vi "practice2_with_strain.vi"() -> ()   [LabVIEW 2014]
doc: "This VI demonstrates the individual configuration of settings in I/W, W/I, and continuous operation modes.\n\nThis VI is not meant to be used with infusion-only models. \n\nNotes:\n(1) If continuous mode is selected, infuse volumes/rates will be used."
uses:
  <instrlib>/KD Scientific 2XX Series/KD Scientific 2XX Series.lvlib
  <vilib>/Motion/FlexMotion/CustomControls/CustomControls.llb/AxisOrVectorSpace To Configure.flx
  <vilib>/Motion/FlexMotion/FunctionsVIs/Trajectory.llb/Check Move Complete Status (8 axes).flx
  <vilib>/Motion/FlexMotion/FunctionsVIs/StartStopMotion.llb/Start Motion (8 axes).flx
  <vilib>/Motion/FlexMotion/FunctionsVIs/StartStopMotion.llb/Stop Motion (8 axes).flx
  <vilib>/vision/NI_Vision_Development_Module.lvlib
panel:
  out "Strain 2 %":dbl
  out "Strain 1 %":dbl
  in  "Distance 2":dbl
  in  "Distance 1":dbl
  out "d 2":i32
  out "d 1":i32
  out "Circle 3":T1
  out "Circle 2":T1
  out "Circle 1":T1
  out "Circles Data (Circle Detection 1)":T2(array[cluster])
  in  "stop (F)":bool
  out "Data from Transducer":dynamicdata(graph) caption="Voltage from Transducer V"
  out "Voltage from pressure transducer":dbl[](array[numeric])
  out "Pressure mm Hg":dbl[](graph)
  in  "Calibration factor":dbl[](array[numeric])
  in  "Zero Error":dbl[](array[numeric])
  out "pressure mm Hg":dbl[](array[numeric])
  in  "stop 2":bool
  out "Voltage (V)":dbl=0.3869919147841388
  out "Force (grams)":dbl=0.3869919147841388
  out "Force Graph (g)":dynamicdata(graph)
  in  "Zero":dbl=-99.6 format="%#_13g"
  out "Load Cell Output (mV)":dynamicdata(graph)
  in  "Displacement in mm":dbl
  in  "Velocity in mm/s":dbl
  out "Image":T3(plugin-control)
  out "Particle Measurements (Pixels) (Particle Analysis 1)":dbl[][](array[numeric]) format="%.2f"
  out "subarray":dbl[](array[numeric])
  out "The diameter":dbl[](array[numeric])
  out "Image from  Vision Acquisition 1":T3(plugin-control)
  out "Units":string
  out "Delivered Volume":dbl
  in  "stop":bool
  out "Status":T4
  in  "Baud Rate (9600)":u32(ring)=9600 items=["300"=300, "1200"=1200, "2400"=2400, "4800"=4800, "9600"=9600]
  in  "Withdrawal Settings":T5={"Flow Rate (5)"=5.0, "Volume (10)"=10.0, "Volume Units (ml)"=enum."milliliters (ml)", "Rate Units (ml/min.)"=enum."milliliters per minute (ml/min.)"} {"Volume (10)" format="%#.3g"}
  in  "Diameter (8.75 mm)":dbl=8.75
  in  "Infusion Settings":T5={"Flow Rate (5)"=5.0, "Volume (10)"=10.0, "Volume Units (ml)"=enum."milliliters (ml)", "Rate Units (ml/min.)"=enum."milliliters per minute (ml/min.)"}
  in  "Operation Mode (Infuse)":u16(ring) items=["Infuse", "Withdraw", "Infuse-Withdraw", "Withdraw-Infuse", "Continuous"]
  in  "Address (0)":i32 format="%0.0f"
  in  "error in (no error)":errorcluster
  in  "VISA resource name":refnum<visa-resource-name>="COM1"
  # "CCD Camera Input"
  # "Load Cell Input"
  # "Syringe Pump Control"
  # "RS-232 Settings"
  # "General Settings"
  # "Pump Status"
  # "Displacement Motor Control"
  # "Pressure Transducer"
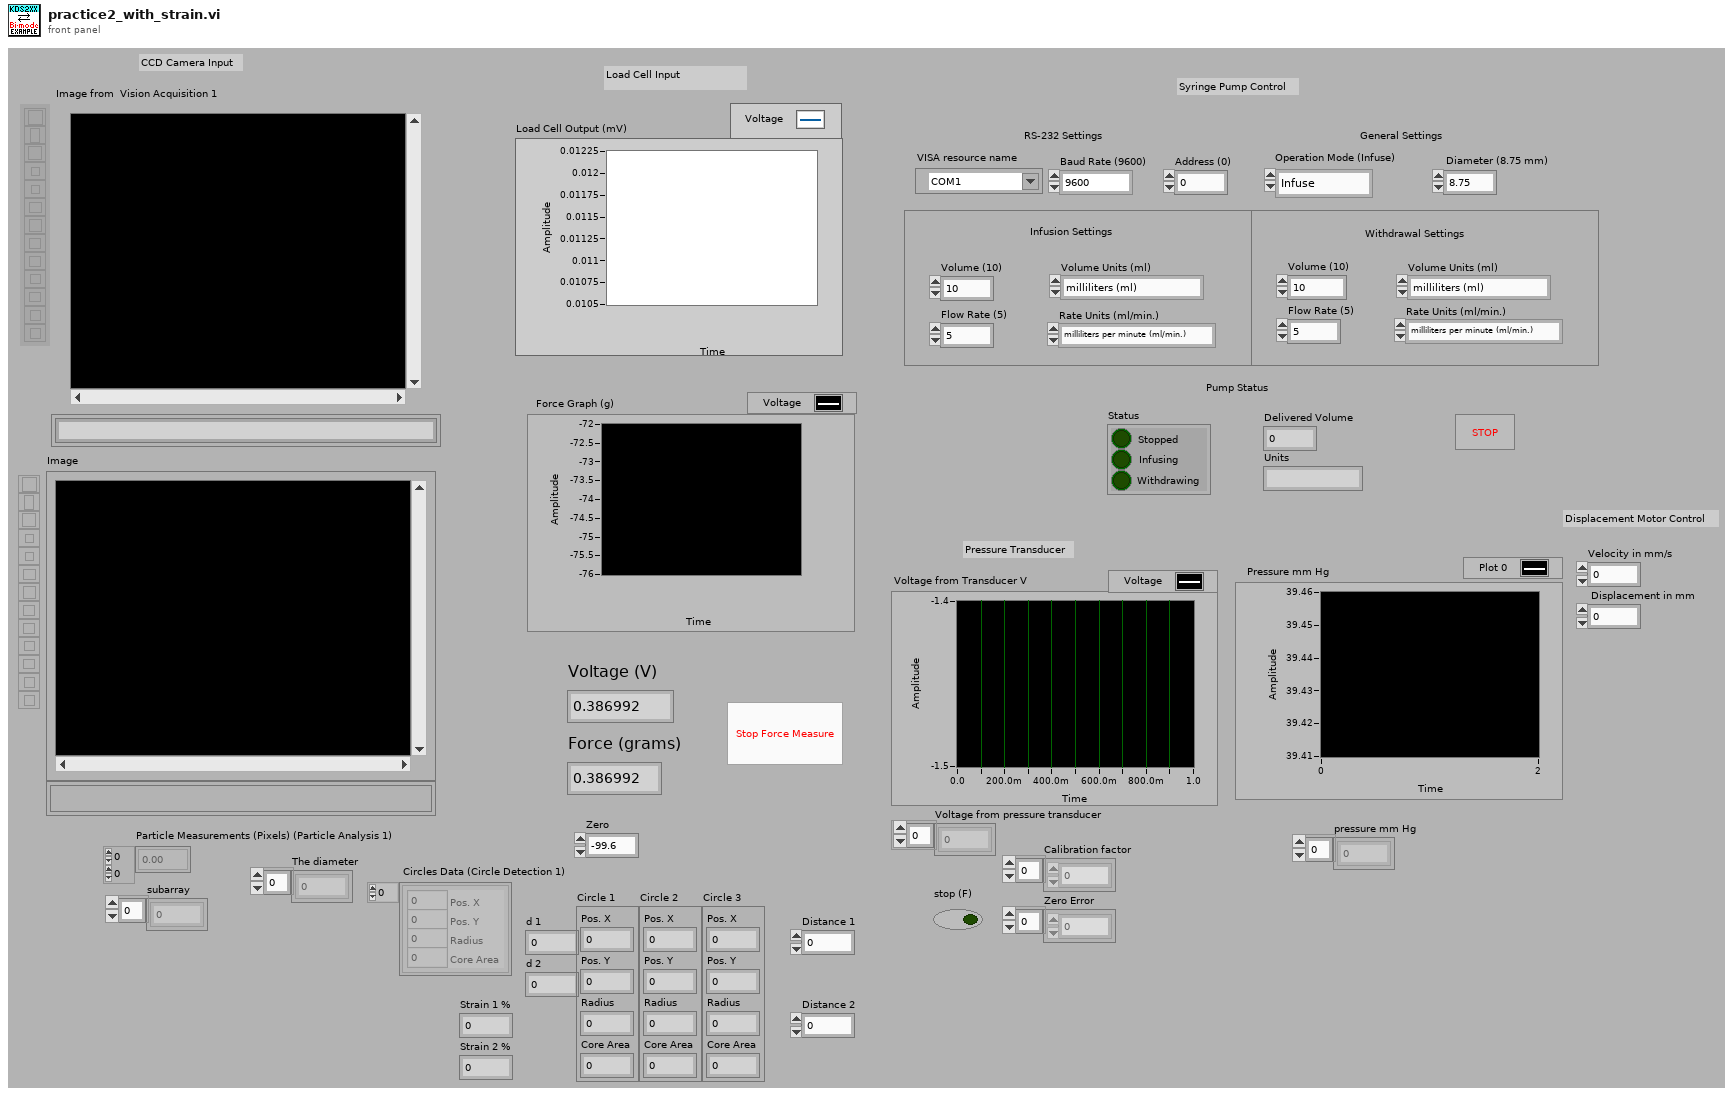
[diagram p1: front panel]
types:
  T1 = cluster{"Pos. X":i32, "Pos. Y":i32, "Radius":i32, "Core Area":i32}
  T2 = cluster{"Pos. X":i32, "Pos. Y":i32, "Radius":i32, "Core Area":i32}[]
  T3 = typedef "IMAQ Image.ctl" = refnum<image>
  T4 = cluster{"Stopped":bool, "Infusing":bool, "Withdrawing":bool}
  T5 = cluster{"Flow Rate (5)":dbl, "Volume (10)":dbl, "Volume Units (ml)":enum16{"milliliters (ml)", "microliters (ul)"}, "Rate Units (ml/min.)":enum16{"milliliters per minute (ml/min.)", "milliliters per hour (ml/hr.)", "microliters per minute (ul/min.)", "microliters per hour (ul/hr.)"}}
  T6 = typedef "Board Id" = u8
  T7 = enum16{"Absolute Position", "Relative Position", "Velocity", "Relative to Cap Pos", "Modulus Position", "Absolute Contouring", "Relative Contouring"}
  T8 = typedef "ROI Descriptor" = cluster{"Global Rectangle":i32[], "Contours":cluster{"ID":enum32{"External", "Internal"}, "Type":u32, "Coordinates":i32[]}[]}
  T9 = typedef "AxisOrVectorSpace To Configure.flx" = u16
  T10 = typedef "Resource Out (Enum).flx" = u16
  T11 = typedef "Bd Id Out" = u8
  T12 = enum16{"milliliters per minute (ml/min.)", "milliliters per hour (ml/hr.)", "microliters per minute (ul/min.)", "microliters per hour (ul/hr.)"}
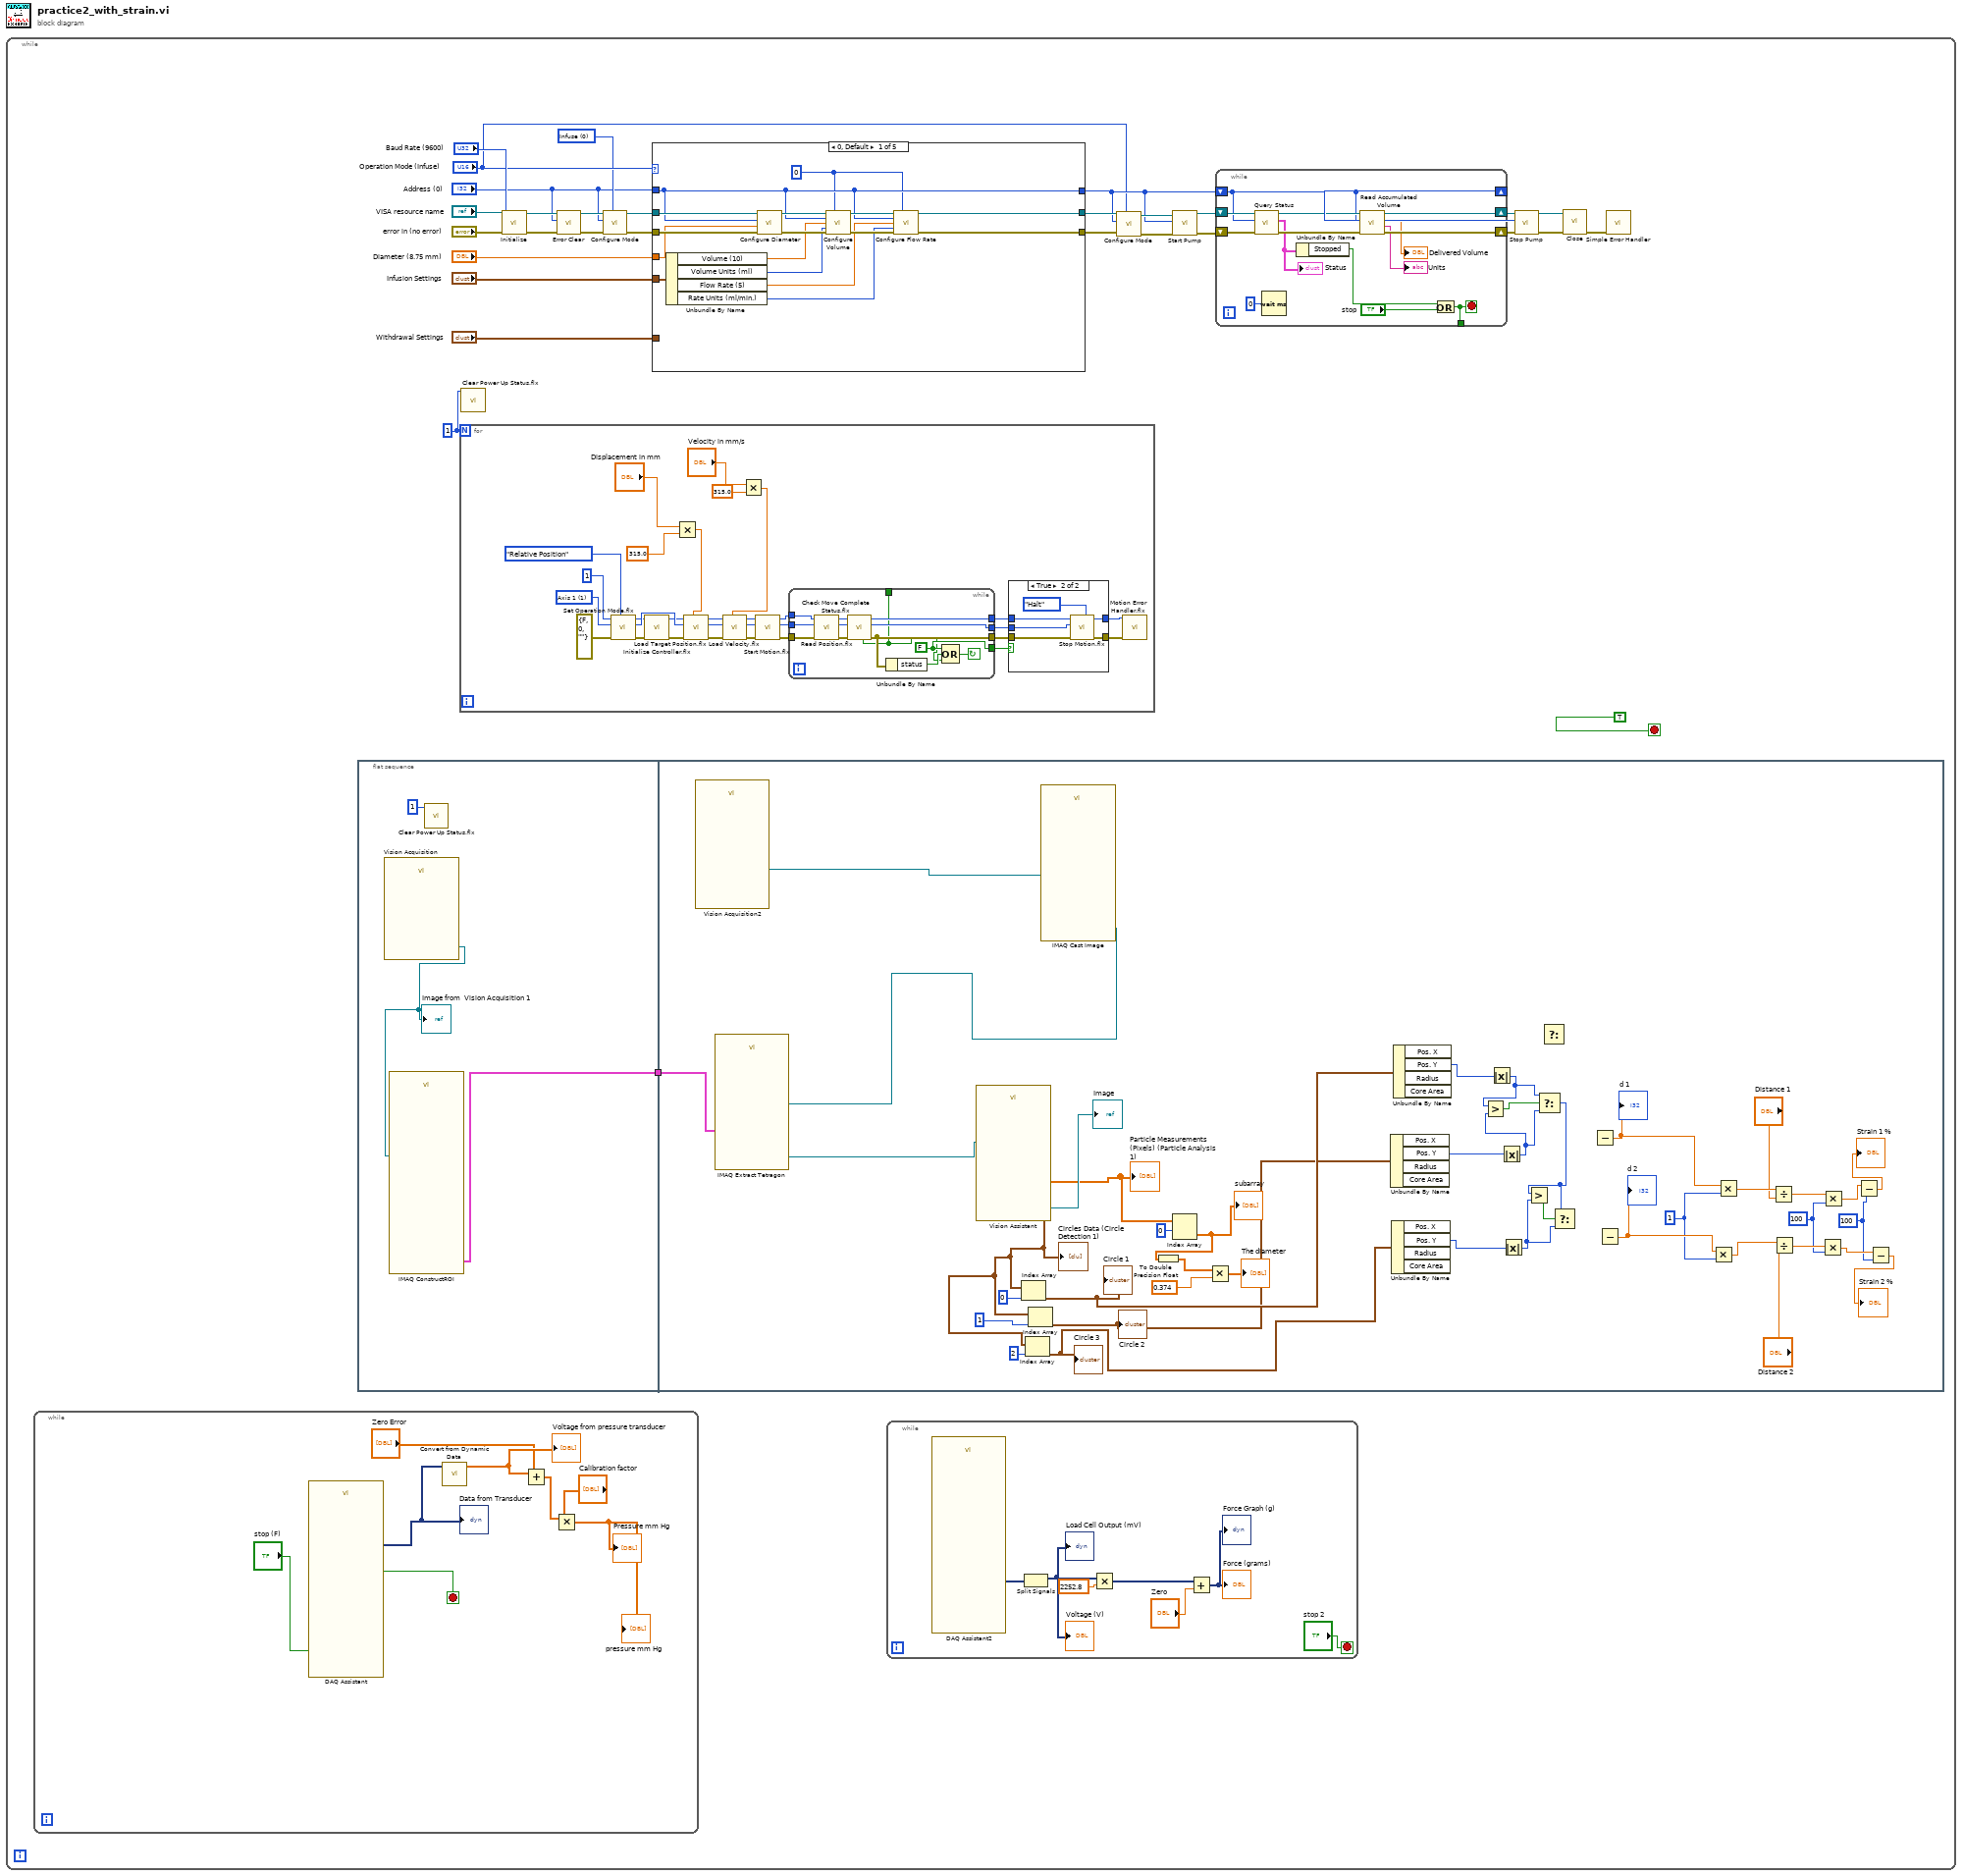
[diagram p0: block diagram]
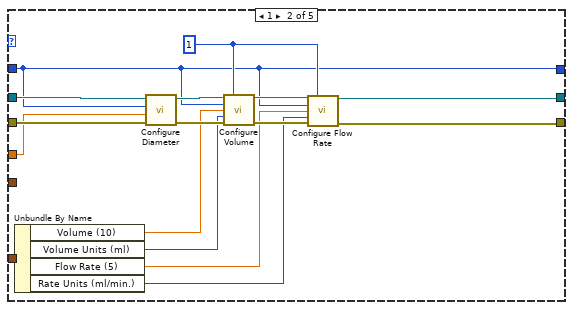
[diagram p3: hidden frame]
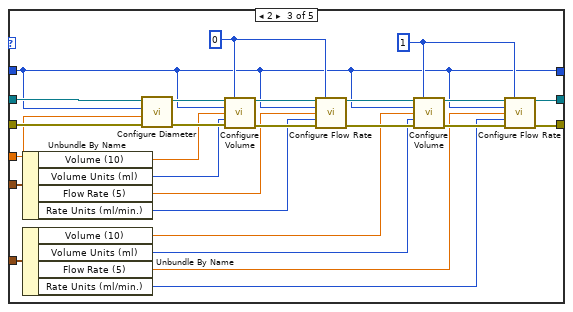
[diagram p4: hidden frame]
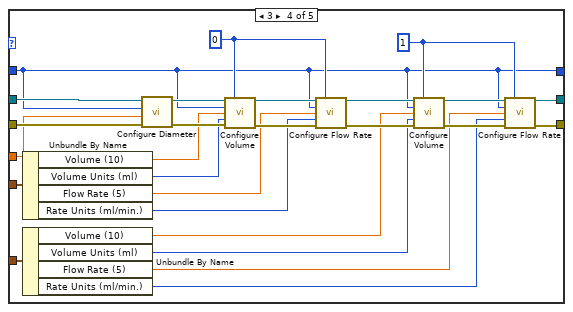
[diagram p5: hidden frame]
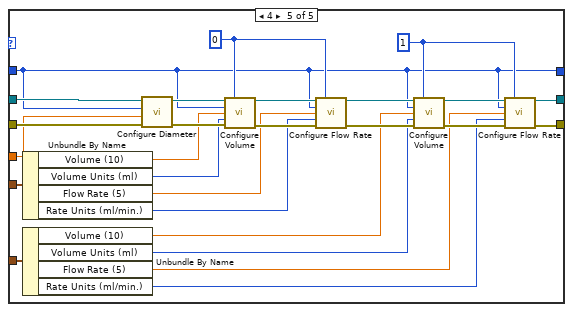
[diagram p6: hidden frame]
diagram:
  n1 = while {
    stop <- TRUE stop-if-true
    w3 = T6 1 ("Board ID")
    w9 = u16 0 items=["Infuse", "Withdraw", "Infuse-Withdraw", "Withdraw-Infuse", "Continuous"] ("Mode (infuse)")
    n2 = flat-sequence {
      tunnel: [w41] -> w1
      tunnel: w1 -> [w83]
      frame #0 {
        n3 = call "Vision Acquisition"() -> ("Image Out"=w39:T3)  [unwired: 26 in, 1 out]
        "Image from  Vision Acquisition 1" <- w39
        n4 = call "IMAQ ConstructROI"("Image"=w39) -> ("ROI Descriptor Out"=w41:T8)  [unwired: 7 in, 3 out]
        n5 = call <vilib>:"Clear Power Up Status.flx"("Board ID"=T6 1) -> ()  [unwired: 6 in, 2 out]
      }
      frame #1 {
        w53 = 100
        w56 = 100
        w63 = 1
        n6 = call "Vision Acquisition2"() -> ("Image Out"=w81:T3)  [unwired: 25 in, 2 out]
        n7 = call "IMAQ Cast Image"("Image Src"=w81) -> ("Image Dst Out"=w80:T3)  [unwired: 9 in, 1 out]
        n8 = call-poly "IMAQ Extract Tetragon"("ROI Descriptor"=w83, "Image Src"=w80) -> ("Image Dst Out"=w73:T3)  [unwired: 8 in, 1 out]
        n9 = call "Vision Assistant"("Image In"=w73) -> ("Image Out"=→"Image":T3, "Particle Measurements (Pixels) (Particle Analysis 1)"=w79:dbl[][], "Circles Data (Circle Detection 1)"=w70:T2)  [unwired: 22 in, 2 out]
        "Particle Measurements (Pixels) (Particle Analysis 1)" <- w79
        "Circles Data (Circle Detection 1)" <- w70
        n10 = Index Array(array=w70, index=0) -> (element=w68:T1)
        "Circle 1" <- w68
        n11 = Index Array(array=w70, index=2) -> (element=w66:T1)
        "Circle 3" <- w66
        n12 = Index Array(array=w70, index=1) -> (element=w67:T1)
        "Circle 2" <- w67
        n13 = Index Array(array=w79, index (row)=0) -> (element=w77:dbl[])  [unwired: 1 in]
        "subarray" <- w77
        n14 = To Double Precision Float(number=w77) -> (double precision float=w76:dbl[])
        n15 = Multiply(x=w76, y=0.374) -> (x*y=→"The diameter":dbl[])
        n16 = Unbundle By Name(w67) -> ("Pos. Y"=w49:i32)  [unwired: 3 out]
        n17 = Unbundle By Name(w66) -> ("Pos. Y"=w48:i32)  [unwired: 3 out]
        n18 = Unbundle By Name(w68) -> ("Pos. Y"=w50:i32)  [unwired: 3 out]
        n19 = Absolute Value(x=w50) -> (abs(x)=w46:i32)
        n20 = Absolute Value(x=w49) -> (abs(x)=w45:i32)
        n21 = Greater?(x=w46, y=w45) -> (0:w47:bool)
        n22 = Absolute Value(x=w48) -> (abs(x)=w42:i32)
        n23 = Select(t=w46, s=w47, f=w45) -> (s? t:f=w43:i32)
        n24 = Greater?(x=w43, y=w42) -> (0:w44:bool)
        n25 = Select() -> ()  [unwired: 3 in, 1 out]
        n26 = Select(t=w43, s=w44, f=w42) -> ()  [unwired: 1 out]
        n27 = Subtract() -> (x-y=w65:dbl)  [unwired: 2 in]
        "d 1" <- w65
        n28 = Subtract() -> (x-y=w64:dbl)  [unwired: 2 in]
        "d 2" <- w64
        n29 = Multiply(x=w64, y=w63) -> (x*y=w61:dbl)
        n30 = Multiply(x=w65, y=w63) -> (x*y=w62:dbl)
        n31 = Divide(x=w62, y="Distance 1") -> (x/y=w58:dbl)
        n32 = Divide(x=w61, y="Distance 2") -> (x/y=w57:dbl)
        n33 = Multiply(x=w57, y=w56) -> (x*y=w54:dbl)
        n34 = Multiply(x=w58, y=w56) -> (x*y=w55:dbl)
        n35 = Subtract(x=w55, y=w53) -> (x-y=→"Strain 1 %":dbl)
        n36 = Subtract(x=w54, y=w53) -> (x-y=→"Strain 2 %":dbl)
      }
    }
    n37 = for {
      N: w3 -> [_]
      w111 = T9 1 items=["Axis 1"=1, "Axis 2"=2, "Axis 3"=3, "Axis 4"=4, "Axis 5"=5, "Axis 6"=6, "Axis 7"=7, "Axis 8"=8, "Vector Space 1"=17, "Vector Space 2"=18, "Vector Space 3"=19, "Vector Space 4"=20] ("Axis or Vector Space")
      n38 = call <vilib>:"Set Operation Mode.flx"("Position Mode (Absolute)"=T7."Relative Position", "error in (no error)"=errorcluster {"status"=FALSE, "code"=0, "source"=""} ("error constant"), "Axis or Vector Space"=w111, "Board ID"=T6 1) -> ("error out"=w109:errorcluster, "Resource Output"=w108:T10, "Bd ID Out"=w107:T11)  [unwired: 2 in]
      n39 = call <vilib>:"Initialize Controller.flx"("error in (no error)"=w109, "Board ID"=w107) -> ("error out"=w102:errorcluster, "Bd ID Out"=w106:T11)  [unwired: 6 in]
      n40 = Multiply(x="Displacement in mm", y=315.0) -> (x*y=w86:dbl)
      n41 = call <vilib>:"Load Target Position.flx"("Target Position (0)"=w86, "error in (no error)"=w102, "Axis"=w108, "Board ID"=w106) -> ("error out"=w103:errorcluster, "Resource Output"=w104:T10, "Bd ID Out"=w105:T11)  [unwired: 3 in]
      n42 = Multiply(x="Velocity in mm/s", y=315.0) -> (x*y=w87:dbl)
      n43 = call <vilib>:"Load Velocity.flx"("Velocity (10000)"=w87, "error in (no error)"=w103, "Axis or Vector Space"=w104, "Board ID"=w105) -> ("error out"=w99:errorcluster, "Resource Output"=w100:T10, "Bd ID Out"=w101:T11)  [unwired: 3 in]
      n44 = call-poly <vilib>:"Start Motion.flx"("error in (no error)"=w99, "Axis or Vector Space"=w100, "Board ID"=w101) -> ("error out"=w96:errorcluster, "Resource Output"=w97:T10, "Bd ID Out"=w98:T11)  [unwired: 3 in]
      n45 = while {
        tunnel: w98 -> [w134]
        tunnel: w97 -> [w133]
        tunnel: w96 -> [w132]
        tunnel: [w127] -> w95
        tunnel: [w126] -> w94
        tunnel: [w124] -> w93
        tunnel: [w123] -> w92
        tunnel: [w122] -> _
        stop <- w128 continue-if-true
        w127 = FALSE
        n46 = call <vilib>:"Read Position.flx"("error in (no error)"=w132, "Axis"=w133, "Board ID"=w134) -> ("error out"=w129:errorcluster, "Resource Output"=w130:T10, "Bd ID Out"=w131:T11)  [unwired: 3 in, 1 out]
        n47 = call-poly <vilib>:"Check Move Complete Status.flx"("error in (no error)"=w129, "Axis or Vector Space"=w130, "Board ID"=w131) -> ("error out"=w126:errorcluster, "Resource Output"=w123:T10, "Bd ID Out"=w124:T11, "Move Complete"=w122:bool)  [unwired: 3 in]
        n48 = Unbundle By Name(w126) -> ("status"=w125:bool)
        n49 = Compound Arithmetic op=OR(w127, w125, w122) -> (w128:bool)
      }
      n50 = case shown="True" w95 {
        tunnel: w94 -> [w114 w120]
        tunnel: w93 -> [w115 w119]
        tunnel: w92 -> [_ w118]
        tunnel: [w114 w117] -> w91
        tunnel: [w115 w116] -> w90
        frame False {
        }
        frame True {
          n51 = call-poly <vilib>:"Stop Motion.flx"("Stop Type (Decel)"=enum16{"Decelerate", "Halt", "Kill"}."Halt", "error in (no error)"=w120, "Axis or Vector Space"=w118, "Board ID"=w119) -> ("error out"=w117:errorcluster, "Bd ID Out"=w116:T11)  [unwired: 3 in, 1 out]
        }
      }
      n52 = call <vilib>:"Motion Error Handler.flx"("Board ID"=w90, "error in (no error)"=w91) -> ()  [unwired: 9 in, 5 out]
    }
    n53 = call <vilib>:"Clear Power Up Status.flx"("Board ID"=w3) -> ()  [unwired: 6 in, 2 out]
    n54 = call <instrlib>:"Initialize.vi"("error in (no error)"="error in (no error)", "Baud Rate (9600)"="Baud Rate (9600)", "VISA resource name"="VISA resource name") -> ("error out"=w6:errorcluster, "VISA resource name out"=w5:refnum<visa-resource-name>)  [unwired: 7 in]
    n55 = call <instrlib>:"Error Clear.vi"("error in (no error)"=w6, "Address (0)"="Address (0)", "VISA resource name"=w5) -> ("error out"=w7:errorcluster, "VISA resource name out"=w8:refnum<visa-resource-name>)  [unwired: 6 in, 1 out]
    n56 = call <instrlib>:"Configure Mode.vi"("Mode (infuse)"=w9, "error in (no error)"=w7, "Address (0)"="Address (0)", "VISA resource name"=w8) -> ("error out"=w11:errorcluster, "VISA resource name out"=w10:refnum<visa-resource-name>)  [unwired: 6 in]
    n57 = case shown="0, Default" "Operation Mode (Infuse)" {
      tunnel: "Infusion Settings" -> [w144 _ w192 w218 w244]
      tunnel: "Withdrawal Settings" -> [_ w166 w191 w217 w243]
      tunnel: w10 -> [w150 w165 w190 w216 w242]
      tunnel: w11 -> [w149 w161 w189 w215 w241]
      tunnel: "Diameter (8.75 mm)" -> [w143 w157 w172 w198 w224]
      tunnel: [w142 w151 w167 w193 w219] -> w13
      tunnel: "Address (0)" -> [w142 w151 w167 w193 w219]
      tunnel: [w137 w162 w169 w195 w221] -> w17
      tunnel: [w136 w158 w168 w194 w220] -> w16
      frame 0, Default {
        w135 = 0
        n58 = Unbundle By Name(w144) -> ("Volume (10)"=w141:dbl, "Volume Units (ml)"=w140:enum16{"milliliters (ml)", "microliters (ul)"}, "Flow Rate (5)"=w139:dbl, "Rate Units (ml/min.)"=w138:T12)
        n59 = call <instrlib>:"Configure Diameter.vi"("error in (no error)"=w149, "Diameter (8.75 mm)"=w143, "Address (0)"=w142, "VISA resource name"=w150) -> ("error out"=w147:errorcluster, "VISA resource name out"=w148:refnum<visa-resource-name>)  [unwired: 6 in]
        n60 = call <instrlib>:"Configure Volume.vi"("VISA resource name"=w148, "Mode (infuse)"=w135, "Address (0)"=w142, "Volume (100)"=w141, "Units (0: milliliters)"=w140, "error in (no error)"=w147) -> ("VISA resource name out"=w146:refnum<visa-resource-name>, "error out"=w145:errorcluster)  [unwired: 8 in]
        n61 = call <instrlib>:"Configure Flow Rate.vi"("VISA resource name"=w146, "Mode (infuse)"=w135, "Address (0)"=w142, "Flow Rate (5)"=w139, "Units (0: milliliters per minute)"=w138, "error in (no error)"=w145) -> ("VISA resource name out"=w137:refnum<visa-resource-name>, "error out"=w136:errorcluster)  [unwired: 8 in]
      }
      frame 1 {
        w152 = 1
        n62 = Unbundle By Name(w166) -> ("Volume (10)"=w156:dbl, "Volume Units (ml)"=w155:enum16{"milliliters (ml)", "microliters (ul)"}, "Flow Rate (5)"=w154:dbl, "Rate Units (ml/min.)"=w153:T12)
        n63 = call <instrlib>:"Configure Diameter.vi"("error in (no error)"=w161, "Diameter (8.75 mm)"=w157, "Address (0)"=w151, "VISA resource name"=w165) -> ("error out"=w160:errorcluster, "VISA resource name out"=w164:refnum<visa-resource-name>)  [unwired: 6 in]
        n64 = call <instrlib>:"Configure Volume.vi"("VISA resource name"=w164, "Mode (infuse)"=w152, "Address (0)"=w151, "Volume (100)"=w156, "Units (0: milliliters)"=w155, "error in (no error)"=w160) -> ("VISA resource name out"=w163:refnum<visa-resource-name>, "error out"=w159:errorcluster)  [unwired: 8 in]
        n65 = call <instrlib>:"Configure Flow Rate.vi"("VISA resource name"=w163, "Mode (infuse)"=w152, "Address (0)"=w151, "Flow Rate (5)"=w154, "Units (0: milliliters per minute)"=w153, "error in (no error)"=w159) -> ("VISA resource name out"=w162:refnum<visa-resource-name>, "error out"=w158:errorcluster)  [unwired: 8 in]
      }
      frame 2 {
        w170 = 1
        w171 = 0
        n66 = Unbundle By Name(w192) -> ("Volume (10)"=w180:dbl, "Volume Units (ml)"=w179:enum16{"milliliters (ml)", "microliters (ul)"}, "Flow Rate (5)"=w178:dbl, "Rate Units (ml/min.)"=w177:T12)
        n67 = Unbundle By Name(w191) -> ("Volume (10)"=w176:dbl, "Volume Units (ml)"=w175:enum16{"milliliters (ml)", "microliters (ul)"}, "Flow Rate (5)"=w174:dbl, "Rate Units (ml/min.)"=w173:T12)
        n68 = call <instrlib>:"Configure Diameter.vi"("error in (no error)"=w189, "Diameter (8.75 mm)"=w172, "Address (0)"=w167, "VISA resource name"=w190) -> ("error out"=w184:errorcluster, "VISA resource name out"=w188:refnum<visa-resource-name>)  [unwired: 6 in]
        n69 = call <instrlib>:"Configure Volume.vi"("VISA resource name"=w188, "Mode (infuse)"=w171, "Address (0)"=w167, "Volume (100)"=w180, "Units (0: milliliters)"=w179, "error in (no error)"=w184) -> ("VISA resource name out"=w187:refnum<visa-resource-name>, "error out"=w183:errorcluster)  [unwired: 8 in]
        n70 = call <instrlib>:"Configure Flow Rate.vi"("VISA resource name"=w187, "Mode (infuse)"=w171, "Address (0)"=w167, "Flow Rate (5)"=w178, "Units (0: milliliters per minute)"=w177, "error in (no error)"=w183) -> ("VISA resource name out"=w186:refnum<visa-resource-name>, "error out"=w182:errorcluster)  [unwired: 8 in]
        n71 = call <instrlib>:"Configure Volume.vi"("VISA resource name"=w186, "Mode (infuse)"=w170, "Address (0)"=w167, "Volume (100)"=w176, "Units (0: milliliters)"=w175, "error in (no error)"=w182) -> ("VISA resource name out"=w185:refnum<visa-resource-name>, "error out"=w181:errorcluster)  [unwired: 8 in]
        n72 = call <instrlib>:"Configure Flow Rate.vi"("VISA resource name"=w185, "Mode (infuse)"=w170, "Address (0)"=w167, "Flow Rate (5)"=w174, "Units (0: milliliters per minute)"=w173, "error in (no error)"=w181) -> ("VISA resource name out"=w169:refnum<visa-resource-name>, "error out"=w168:errorcluster)  [unwired: 8 in]
      }
      frame 3 {
        w196 = 1
        w197 = 0
        n73 = Unbundle By Name(w218) -> ("Volume (10)"=w206:dbl, "Volume Units (ml)"=w205:enum16{"milliliters (ml)", "microliters (ul)"}, "Flow Rate (5)"=w204:dbl, "Rate Units (ml/min.)"=w203:T12)
        n74 = Unbundle By Name(w217) -> ("Volume (10)"=w202:dbl, "Volume Units (ml)"=w201:enum16{"milliliters (ml)", "microliters (ul)"}, "Flow Rate (5)"=w200:dbl, "Rate Units (ml/min.)"=w199:T12)
        n75 = call <instrlib>:"Configure Diameter.vi"("error in (no error)"=w215, "Diameter (8.75 mm)"=w198, "Address (0)"=w193, "VISA resource name"=w216) -> ("error out"=w210:errorcluster, "VISA resource name out"=w214:refnum<visa-resource-name>)  [unwired: 6 in]
        n76 = call <instrlib>:"Configure Volume.vi"("VISA resource name"=w214, "Mode (infuse)"=w197, "Address (0)"=w193, "Volume (100)"=w206, "Units (0: milliliters)"=w205, "error in (no error)"=w210) -> ("VISA resource name out"=w213:refnum<visa-resource-name>, "error out"=w209:errorcluster)  [unwired: 8 in]
        n77 = call <instrlib>:"Configure Flow Rate.vi"("VISA resource name"=w213, "Mode (infuse)"=w197, "Address (0)"=w193, "Flow Rate (5)"=w204, "Units (0: milliliters per minute)"=w203, "error in (no error)"=w209) -> ("VISA resource name out"=w212:refnum<visa-resource-name>, "error out"=w208:errorcluster)  [unwired: 8 in]
        n78 = call <instrlib>:"Configure Volume.vi"("VISA resource name"=w212, "Mode (infuse)"=w196, "Address (0)"=w193, "Volume (100)"=w202, "Units (0: milliliters)"=w201, "error in (no error)"=w208) -> ("VISA resource name out"=w211:refnum<visa-resource-name>, "error out"=w207:errorcluster)  [unwired: 8 in]
        n79 = call <instrlib>:"Configure Flow Rate.vi"("VISA resource name"=w211, "Mode (infuse)"=w196, "Address (0)"=w193, "Flow Rate (5)"=w200, "Units (0: milliliters per minute)"=w199, "error in (no error)"=w207) -> ("VISA resource name out"=w195:refnum<visa-resource-name>, "error out"=w194:errorcluster)  [unwired: 8 in]
      }
      frame 4 {
        w222 = 1
        w223 = 0
        n80 = Unbundle By Name(w244) -> ("Volume (10)"=w232:dbl, "Volume Units (ml)"=w231:enum16{"milliliters (ml)", "microliters (ul)"}, "Flow Rate (5)"=w230:dbl, "Rate Units (ml/min.)"=w229:T12)
        n81 = Unbundle By Name(w243) -> ("Volume (10)"=w228:dbl, "Volume Units (ml)"=w227:enum16{"milliliters (ml)", "microliters (ul)"}, "Flow Rate (5)"=w226:dbl, "Rate Units (ml/min.)"=w225:T12)
        n82 = call <instrlib>:"Configure Diameter.vi"("error in (no error)"=w241, "Diameter (8.75 mm)"=w224, "Address (0)"=w219, "VISA resource name"=w242) -> ("error out"=w236:errorcluster, "VISA resource name out"=w240:refnum<visa-resource-name>)  [unwired: 6 in]
        n83 = call <instrlib>:"Configure Volume.vi"("VISA resource name"=w240, "Mode (infuse)"=w223, "Address (0)"=w219, "Volume (100)"=w232, "Units (0: milliliters)"=w231, "error in (no error)"=w236) -> ("VISA resource name out"=w239:refnum<visa-resource-name>, "error out"=w235:errorcluster)  [unwired: 8 in]
        n84 = call <instrlib>:"Configure Flow Rate.vi"("VISA resource name"=w239, "Mode (infuse)"=w223, "Address (0)"=w219, "Flow Rate (5)"=w230, "Units (0: milliliters per minute)"=w229, "error in (no error)"=w235) -> ("VISA resource name out"=w238:refnum<visa-resource-name>, "error out"=w234:errorcluster)  [unwired: 8 in]
        n85 = call <instrlib>:"Configure Volume.vi"("VISA resource name"=w238, "Mode (infuse)"=w222, "Address (0)"=w219, "Volume (100)"=w228, "Units (0: milliliters)"=w227, "error in (no error)"=w234) -> ("VISA resource name out"=w237:refnum<visa-resource-name>, "error out"=w233:errorcluster)  [unwired: 8 in]
        n86 = call <instrlib>:"Configure Flow Rate.vi"("VISA resource name"=w237, "Mode (infuse)"=w222, "Address (0)"=w219, "Flow Rate (5)"=w226, "Units (0: milliliters per minute)"=w225, "error in (no error)"=w233) -> ("VISA resource name out"=w221:refnum<visa-resource-name>, "error out"=w220:errorcluster)  [unwired: 8 in]
      }
    }
    n87 = while {
      stop <- "stop 2" stop-if-true
      n88 = call "DAQ Assistant2"() -> ("data"=w37:dynamicdata)  [unwired: 16 in, 3 out]
      n89 = Split Signals(w37) -> (w32:dynamicdata)  [unwired: 2 in, 1 out]
      "Voltage (V)" <- w32
      "Load Cell Output (mV)" <- w32
      n90 = Multiply(x=w32, y=2252.8) -> (x*y=w36:dynamicdata)
      n91 = Add(x=w36, y="Zero") -> (x+y=→"Force (grams)" →"Force Graph (g)":dynamicdata)
    }
    n92 = call <instrlib>:"Configure Mode.vi"("Mode (infuse)"="Operation Mode (Infuse)", "error in (no error)"=w16, "Address (0)"=w13, "VISA resource name"=w17) -> ("error out"=w14:errorcluster, "VISA resource name out"=w15:refnum<visa-resource-name>)  [unwired: 6 in]
    n93 = call <instrlib>:"Start Pump.vi"("error in (no error)"=w14, "Address (0)"=w13, "VISA resource name"=w15) -> ("error out"=w28:errorcluster, "VISA resource name out"=w29:refnum<visa-resource-name>)  [unwired: 7 in]
    n94 = while {
      shift-right: [w248] -> w22
      shift-left: w13 -> [w248]
      shift-right: [w250] -> w27
      shift-left: w29 -> [w255]
      shift-right: [w249] -> w26
      shift-left: w28 -> [w256]
      tunnel: [w245] -> _
      stop <- w245 stop-if-true
      n95 = call <instrlib>:"Query Status.vi"("error in (no error)"=w256, "Address (0)"=w248, "VISA resource name"=w255) -> ("error out"=w258:errorcluster, "Status"=w254:T4, "VISA resource name out"=w251:refnum<visa-resource-name>)  [unwired: 6 in]
      "Status" <- w254
      n96 = Wait (ms)(milliseconds to wait=u32 0) -> ()  [unwired: 1 out]
      n97 = Unbundle By Name(w254) -> ("Stopped"=w253:bool)
      n98 = call <instrlib>:"Read Accumulated Volume.vi"("error in (no error)"=w258, "Address (0)"=w248, "VISA resource name"=w251) -> ("error out"=w249:errorcluster, "Units"=→"Units":string, "Delivered Volume"=→"Delivered Volume":dbl, "VISA resource name out"=w250:refnum<visa-resource-name>)  [unwired: 5 in]
      n99 = Or(x=w253, y="stop") -> (x .or. y?=w245:bool)
    }
    n100 = call <instrlib>:"Stop Pump.vi"("error in (no error)"=w26, "Address (0)"=w22, "VISA resource name"=w27) -> ("error out"=w20:errorcluster, "VISA resource name out"=w19:refnum<visa-resource-name>)  [unwired: 7 in]
    n101 = call <instrlib>:"Close.vi"("error in (no error)"=w20, "VISA resource name"=w19) -> ("error out"=w21:errorcluster)  [unwired: 9 in]
    n102 = call <vilib>:"Simple Error Handler.vi"("error in (no error)"=w21) -> ()  [unwired: 4 in, 5 out]
  }
  n103 = while {
    stop <- w265 stop-if-true
    n104 = call "DAQ Assistant"("stop (F)"="stop (F)") -> ("data"=w264:dynamicdata, "stopped"=w265:bool)  [unwired: 15 in, 2 out]
    "Data from Transducer" <- w264
    n105 = call "Convert from Dynamic Data"("Dynamic Data Type"=w264) -> ("Array"=w261:dbl[])  [unwired: 3 in]
    "Voltage from pressure transducer" <- w261
    n106 = Add(x=w261, y="Zero Error") -> (x+y=w259:dbl[])
    n107 = Multiply(x=w259, y="Calibration factor") -> (x*y=→"Pressure mm Hg" →"pressure mm Hg":dbl[])
  }
